vi "Find ODBC driver from registry.vi"(8 "error in (no error)":errorcluster) -> (0 "error out":errorcluster, 2 "driver":string)   [LabVIEW 2018]
uses:
  <vilib>/registry/registry.llb/Registry View.ctl
  <vilib>/registry/registry.llb/Registry RtKey.ctl
  <vilib>/registry/registry.llb/Registry SAM.ctl
panel:
  out "values":string[](array[string])
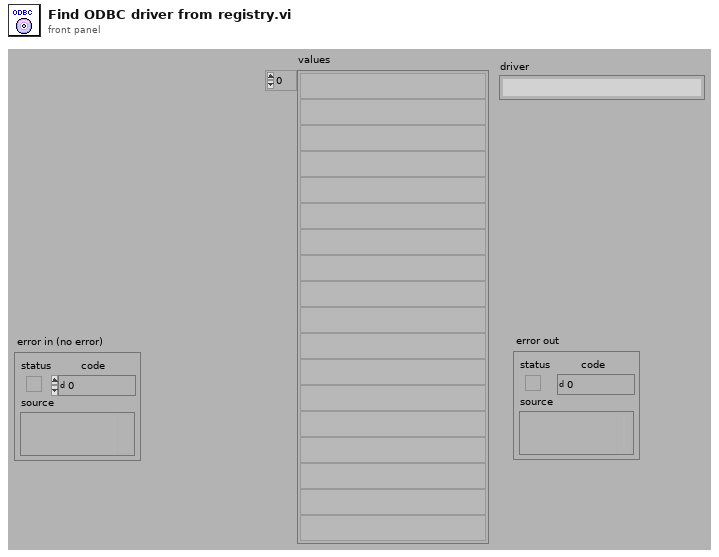
[diagram p1: front panel]
types:
  T1 = typedef "Registry SAM.ctl" = enum32{"KEY_QUERY_VALUE", "KEY_SET_VALUE", "KEY_CREATE_SUB_KEY", "KEY_ENUMERATE_SUB_KEYS", "KEY_NOTIFY", "KEY_CREATE_LINK", "KEY_READ", "KEY_WRITE", "KEY_ALL_ACCESS", "KEY_READ | KEY_WRITE"}
  T2 = typedef "Registry RtKey.ctl" = enum32{"HKEY_CLASSES_ROOT", "HKEY_CURRENT_USER", "HKEY_LOCAL_MACHINE", "HKEY_USERS", "HKEY_PERFORMANCE_DATA", "HKEY_CURRENT_CONFIG", "HKEY_DYN_DATA"}
  T3 = typedef "Registry View.ctl" = u16
  T4 = typedef "Registry refnum.ctl" = refnum<k1>
  T5 = cluster{"numValues":i32, "maxValueNameLen":i32, "maxValueDataLen":i32}
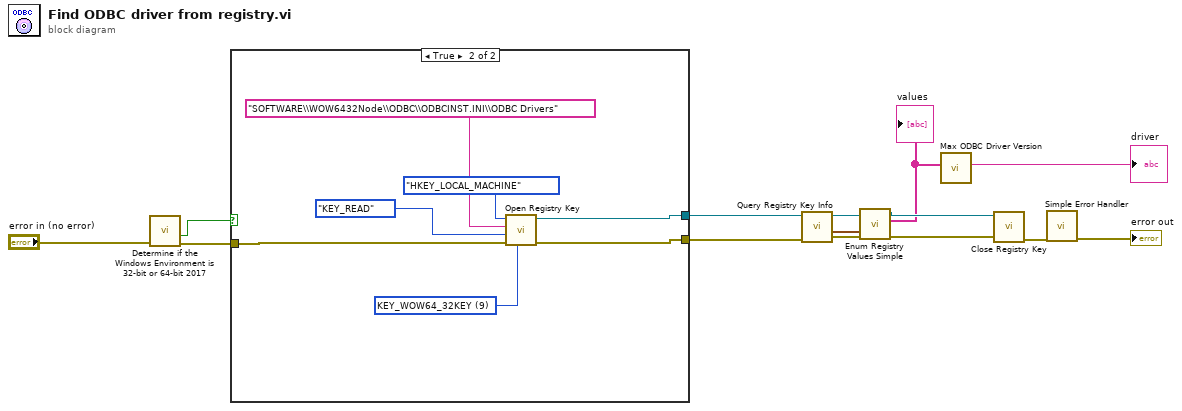
[diagram p0: block diagram]
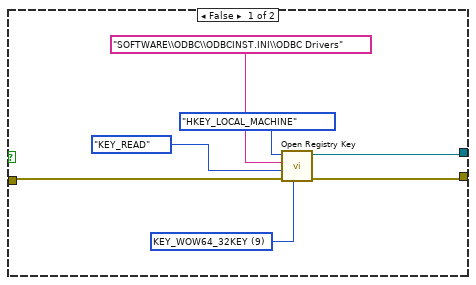
[diagram p2: hidden frame]
diagram:
  n1 = call "Determine if the Windows Environment is 32-bit or 64-bit 2017.vi"("error in"="error in (no error)") -> ("error out"=w2:errorcluster, "64-bit system"=w1:bool)  [unwired: 9 in]
  n2 = case shown="True" w1 {
    tunnel: [w16 w24] -> w12
    tunnel: [w15 w23] -> w11
    tunnel: w2 -> [w17 w22]
    frame False {
      w19 = T3 9 items=["Default"=0, "KEY_WOW64_64KEY"=8, "KEY_WOW64_32KEY"=9] ("registry view")
      n3 = call <vilib>:"Open Registry Key.vi"("registry view"=w19, "error in (no error)"=w17, "security access mask (KEY_READ | KEY_WRITE)"=Registry_SAM."KEY_READ", "subkey"="SOFTWARE\\ODBC\\ODBCINST.INI\\ODBC Drivers", "root key (HKEY_LOCAL_MACHINE)"=Registry_RtKey."HKEY_LOCAL_MACHINE") -> ("error out"=w16:errorcluster, "refnum out"=w15:T4)  [unwired: 5 in]
    }
    frame True {
      w26 = T3 9 items=["Default"=0, "KEY_WOW64_64KEY"=8, "KEY_WOW64_32KEY"=9] ("registry view")
      n4 = call <vilib>:"Open Registry Key.vi"("registry view"=w26, "error in (no error)"=w22, "security access mask (KEY_READ | KEY_WRITE)"=Registry_SAM."KEY_READ", "subkey"="SOFTWARE\\WOW6432Node\\ODBC\\ODBCINST.INI\\ODBC Drivers", "root key (HKEY_LOCAL_MACHINE)"=Registry_RtKey."HKEY_LOCAL_MACHINE") -> ("error out"=w24:errorcluster, "refnum out"=w23:T4)  [unwired: 5 in]
    }
  }
  n5 = call <vilib>:"Query Registry Key Info.vi"("error in (no error)"=w12, "refnum"=w11) -> ("error out"=w7:errorcluster, "value info"=w6:T5, "refnum out"=w8:T4)  [unwired: 5 in, 2 out]
  n6 = call <vilib>:"Enum Registry Values Simple.vi"("error in (no error)"=w7, "value info"=w6, "refnum"=w8) -> ("error out"=w9:errorcluster, "values"=w5:string[], "refnum out"=w10:T4)  [unwired: 3 in, 3 out]
  "values" <- w5
  n7 = call "Max ODBC Driver Version.vi"("Drivers"=w5) -> ("driver"=→"driver":string)  [unwired: 10 in]
  n8 = call <vilib>:"Close Registry Key.vi"("error in (no error)"=w9, "refnum"=w10) -> ("error out"=w14:errorcluster)  [unwired: 5 in]
  n9 = call <vilib>:"Simple Error Handler.vi"("error in (no error)"=w14) -> ("error out"=→"error out":errorcluster)  [unwired: 4 in, 4 out]
